vi "VI-Layout XControl State.vi"(0 "Path":path=path "C:/Users/hancock/Desktop/Test/Test.xctl", 11 "error in (no error)":errorcluster) -> (15 "error out":errorcluster)   [LabVIEW 2015]
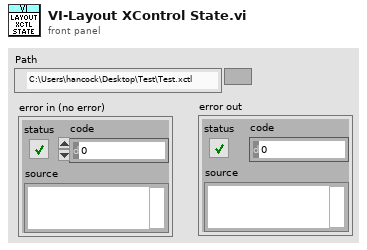
[diagram p1: front panel]
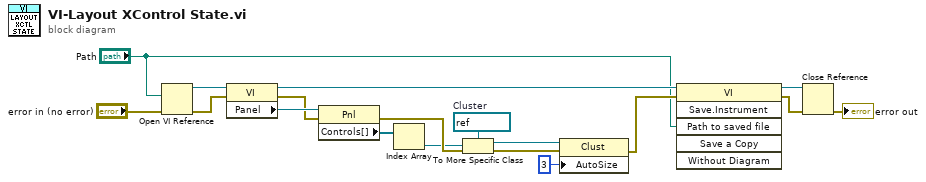
[diagram p0: block diagram]
diagram:
  w17 = refnum<vi> refnum  # Cluster
  n1 = Open VI Reference(vi path="Path", error in (no error)="error in (no error)") -> (vi reference=w8:refnum<vi>, error out=w11:errorcluster)  [unwired: 4 in]
  n2 = property class="VI"(reference=w8, error in=w11) -> (reference out=w7:refnum<vi>, error out=w13:errorcluster, "Panel"=w14:refnum<vi>)
  n3 = property class="Pnl"(reference=w14, error in=w13) -> (error out=w18:errorcluster, "Controls[]"=w15:refnum<vi>[])  [unwired: 1 out]
  n4 = Index Array(array=w15) -> (element=w16:refnum<vi>)  [unwired: 1 in]
  n5 = To More Specific Class(target class=w17, reference=w16, error in=w18) -> (specific class reference=w10:refnum<vi>, error out=w9:errorcluster)
  n6 = property class="Clust"(reference=w10, error in=w9, "AutoSize"=u32 3 ("Auto Sizing")) -> (error out=w3:errorcluster)  [unwired: 1 out]
  n7 = invoke class="VI" method="Save.Instrument"(reference=w7, error in=w3, "Path to saved file"="Path") -> (reference out=w4:refnum<vi>, error out=w2:errorcluster)  [unwired: 3 in, 4 out]
  n8 = Close Reference(reference=w4, error in (no error)=w2) -> (error out=→"error out":errorcluster)
